vi "mao01.vi"   [LabVIEW 2014]
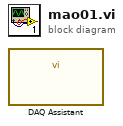
[diagram p0: block diagram]
diagram:
  n1 = call "DAQ Assistant"() -> ()  [unwired: 12 in]
